vi "enumerateStaticDependencies.vi"(8 "error in (no error)":errorcluster, 11 "SMO.SelfTerminatingOverride":refnum<class "SMO.SelfTerminatingOverride.lvclass">) -> (0 "error out":errorcluster, 2 "Static Dependencies":refnum<class "Dependency.lvclass">[](array[class]), 3 "SMO.SelfTerminatingOverride out":refnum<class "SMO.SelfTerminatingOverride.lvclass">)   [LabVIEW 2013, in "SMO.SelfTerminatingOverride.lvclass"]
uses:
  SMO.SelfTerminatingOverride.lvclass
  Dependency/Dependency.lvclass
  SMO/SMO.lvclass
  SMO.SelfTerminating/SMO.SelfTerminating.lvclass
panel:
  # "For instructions on how to use the JKI State Machine Objects, examples and video tutorials, visit:\nhttp://jki.net/state-machine-objects/\n\nJKI State Machine Objects™\nhttp://jki.net/state-machine-objects/\nCopyright (C) 2005-2015, JKI <info@jki.net>\nALL RIGHTS RESERVED"
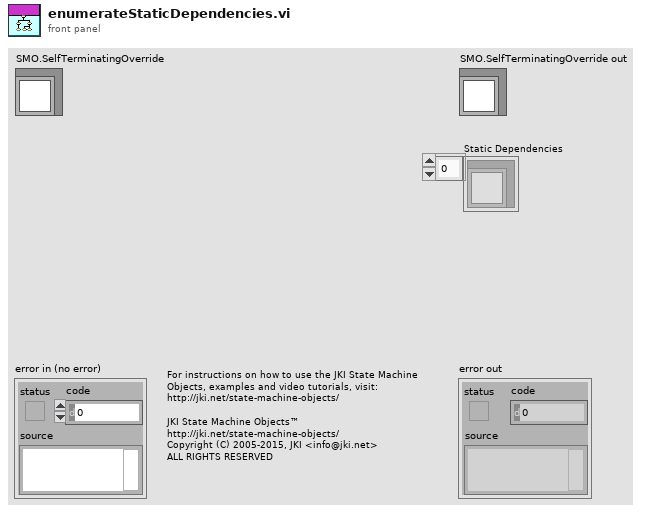
[diagram p1: front panel]
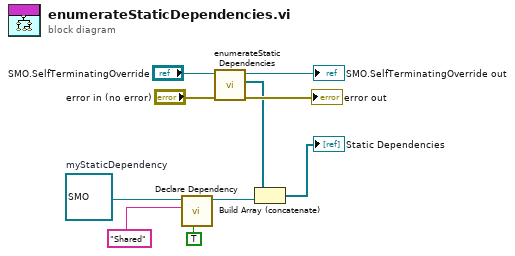
[diagram p0: block diagram]
diagram:
  w6 = refnum<class "SMO.lvclass"> refnum  # myStaticDependency
  n1 = call "Declare Dependency.vi"("Shared Resource (F)"=TRUE, "Name"="Shared", "Type"=w6) -> ("Dependency out"=w3:refnum<class "Dependency.lvclass">)  [unwired: 7 in, 1 out]
  n2 = call-parent "enumerateStaticDependencies.vi"("error in (no error)"="error in (no error)", "SMO"="SMO.SelfTerminatingOverride") -> ("error out"=→"error out":errorcluster, "Static Dependencies"=w2:refnum<class "Dependency.lvclass">[], "SMO out"=→"SMO.SelfTerminatingOverride out":refnum<class "SMO.SelfTerminatingOverride.lvclass">)  [unwired: 7 in]
  n3 = Build Array (concatenate)(w2, w3) -> (→"Static Dependencies":refnum<class "Dependency.lvclass">[])
